vi "AllConnect Status update.vi"(8 "error in (no error)":errorcluster, 11 "Control-Client in":refnum<class "Control-Client.lvclass">) -> (0 "error out":errorcluster, 3 "Control-Client out":refnum<class "Control-Client.lvclass">)   [LabVIEW 2015, in "Control-Client.lvclass"]
uses:
  Control-Client.lvclass
  Control-Client.lvclass/Control-Client.ctl
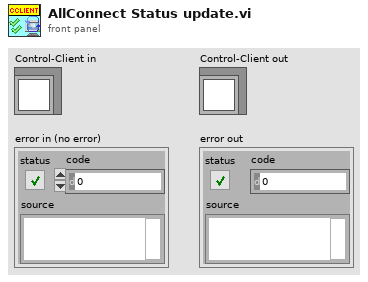
[diagram p1: front panel]
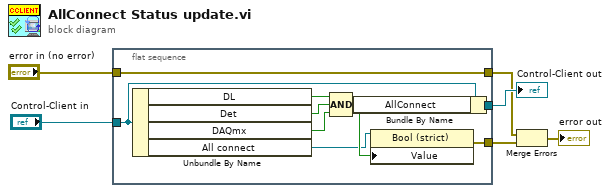
[diagram p0: block diagram]
diagram:
  n1 = flat-sequence {
    tunnel: [w15] -> w3
    tunnel: [w9] -> w6
    tunnel: "Control-Client in" -> [w8]
    tunnel: [w7] -> w2
    tunnel: "error in (no error)" -> [w7]
    frame #0 {
      n2 = Unbundle By Name(w8) -> ("DL"=w10:bool, "Det"=w11:bool, "DAQmx"=w12:bool, "All connect"=w13:refnum<vi>)
      n3 = Compound Arithmetic op=AND(w10, w11, w12) -> (w14:bool)
      n4 = Bundle By Name(cluster=w8, "AllConnect"=w14) -> (w9:refnum<class "Control-Client.lvclass">)
      n5 = property class="Bool (strict)"(reference=w13, "Value"=w14) -> (error out=w15:errorcluster)  [unwired: 1 in, 1 out]
    }
  }
  n6 = Merge Errors(w2, w3) -> (→"error out":errorcluster)
  "Control-Client out" <- w6
